vi "major_buff.vi"(2 "Кол-во копий":i32=5, 3 "Размер окна":i32=4, 4 "Биты на выходе 1":dbl[](array[numeric])) -> (0 "Подготовленный к отправке мажоритарный код":dbl[][](array[numeric]), 1 "2-х массив на выходе 3":dbl[][](array[numeric]))   [LabVIEW 2013]
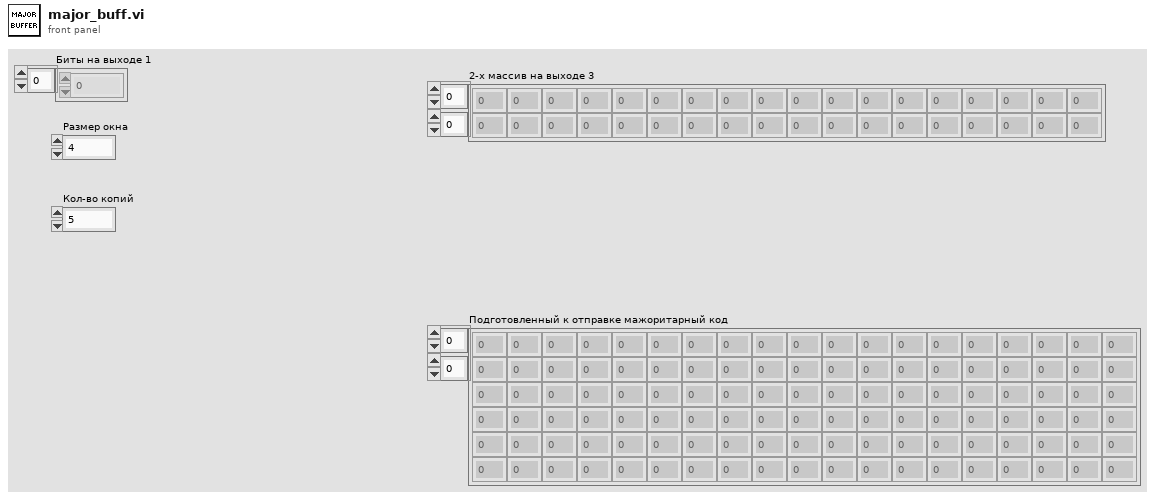
[diagram p1: front panel]
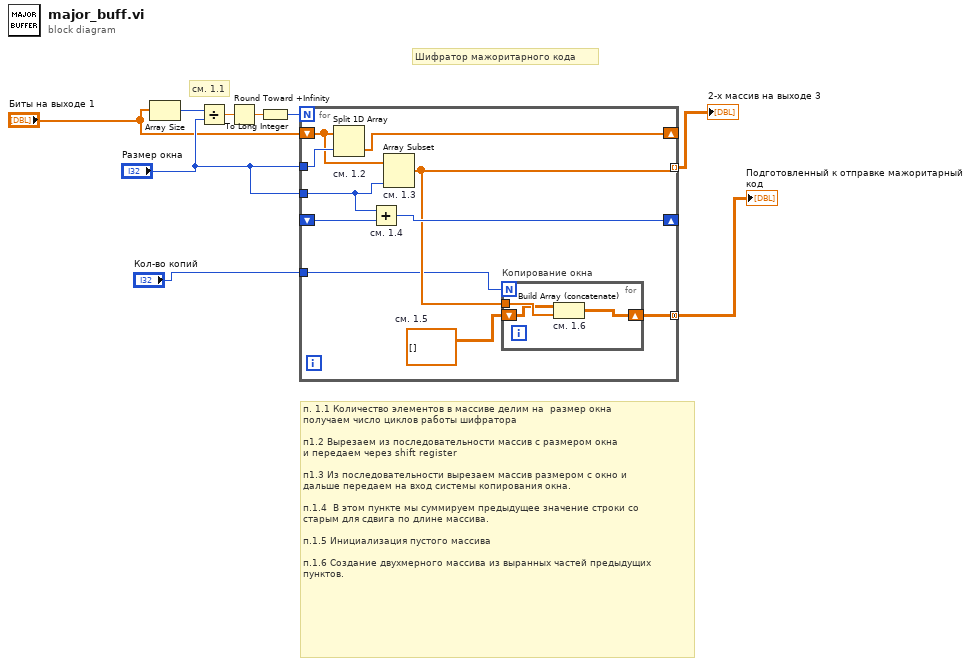
[diagram p0: block diagram]
diagram:
  # "п. 1.1 Количество элементов в массиве делим на  размер окна\nполучаем число циклов работы шифратора\n\nп1.2 Вырезаем из последовательности массив с размером окна \nи передаем через shift register\n\nп1.3 Из последовательности вырезаем массив размером с окно и \nдальше передаем на вход системы копирования окна.\n \nп.1.4  В этом пункте мы суммируем предыдущее значение строки со\nстарым для сдвига по длине массива.\n\nп.1.5 Инициализация пустого массива\n\nп.1.6 Создание двухмерного массива из выранных частей предыдущих\nпунктов."
  # "см. 1.1"
  # "Шифратор мажоритарного кода"
  n1 = Array Size(array="Биты на выходе 1") -> (size(s)=w9:i32)
  n2 = Divide(x=w9, y="Размер окна") -> (x/y=w8:dbl)
  n3 = Round Toward +Infinity(x=w8) -> (ceil(x): smallest int >= x=w7:dbl)
  n4 = To Long Integer(number=w7) -> (32bit integer=w4:i32)
  n5 = for {
    N: w4 -> [_]
    shift-right: [w19] -> _
    shift-left: "Биты на выходе 1" -> [w17]
    tunnel: "Размер окна" -> [w18]
    shift-right: [w15] -> _
    shift-left: _ -> [w14]
    tunnel: "Размер окна" -> [w16]
    tunnel: [w13] -> w5 mode=indexing
    tunnel: [w12] -> w3 mode=concatenating
    tunnel: "Кол-во копий" -> [w10]
    w11 = dbl[][] []  # см. 1.5
    n6 = Split 1D Array "см. 1.2"(array=w17, index=w18) -> (second subarray=w19:dbl[])  [unwired: 1 out]
    n7 = Add "см. 1.4"(x=w16, y=w14) -> (x+y=w15:i32)
    n8 = Array Subset "см. 1.3"(array=w17, length=w16) -> (w13:dbl[])  [unwired: 1 in]
    n9 = for "Копирование окна" {
      N: w10 -> [_]
      tunnel: w13 -> [w21]
      shift-right: [w22] -> w12
      shift-left: w11 -> [w20]
      n10 = Build Array (concatenate) "см. 1.6"(w20, w21) -> (w22:dbl[][])
    }
  }
  "2-х массив на выходе 3" <- w5
  "Подготовленный к отправке мажоритарный код" <- w3
